vi "PID controlled cooling fan system.vi"() -> ()   [LabVIEW 2024]
panel:
  out "Waveform Chart":cluster{"Temperature (C)":dbl, u8, u8}(graph)
  out "Fan Speed RPM":dbl
  in  "Hardware":bool
  in  "K_d":dbl
  in  "K_i":dbl
  in  "K_p":dbl
  in  "Temperature (C)":dbl
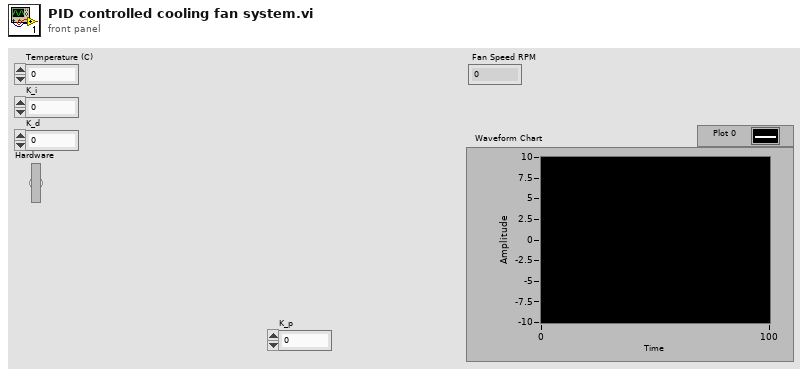
[diagram p1: front panel]
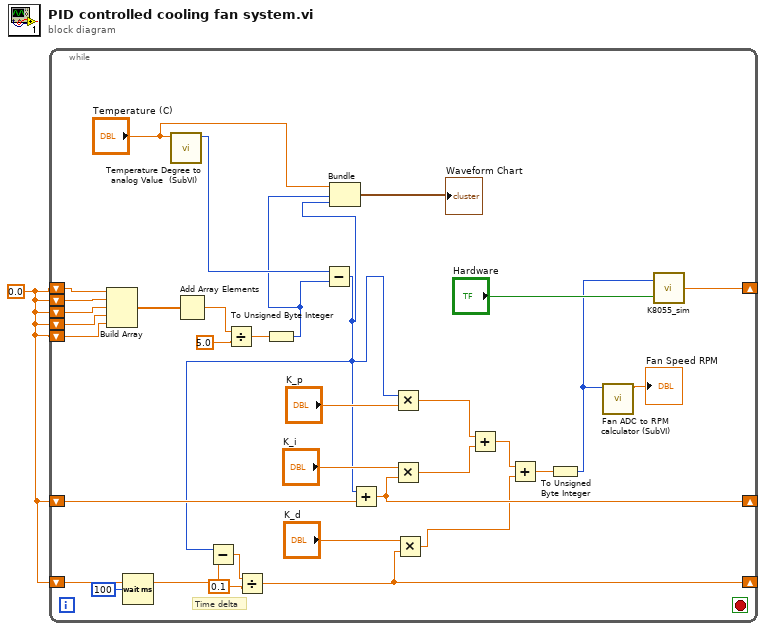
[diagram p0: block diagram]
diagram:
  w1 = 0.0 ("Read temp")
  n1 = while {
    shift-right: [w29] -> _
    shift-left: w1 -> [w34]
    shift-left: w1 -> [w30]
    shift-left: w1 -> [w33]
    shift-left: w1 -> [w32]
    shift-left: w1 -> [w31]
    shift-right: [w19] -> _
    shift-left: w1 -> [w20]
    shift-right: [w6] -> _
    shift-left: w1 -> [w14]
    stop <- _ stop-if-true
    # "Time delta"
    n2 = Build Array(w34, w33, w32, w31, w30) -> (w28:dbl[])
    n3 = Wait (ms)(milliseconds to wait=u32 100) -> ()  [unwired: 1 out]
    n4 = call "Temperature Degree to analog Value  (SubVI).vi"("Temperature (C)"="Temperature (C)") -> ("Temperature Analog Value"=w24:u8)  [unwired: 10 in]
    n5 = Add Array Elements(numeric array=w28) -> (sum=w26:dbl)
    n6 = Divide(x=w26, y=5.0) -> (x/y=w25:dbl)
    n7 = To Unsigned Byte Integer(number=w25) -> (unsigned 8bit integer=w5:u8)
    n8 = Subtract(x=w24, y=w5) -> (x-y=w3:u8)
    n9 = Subtract(x=w3, y=w14) -> (x-y=w13:dbl)
    n10 = Divide(x=w13, y=0.1) -> (x/y=w6:dbl)
    n11 = Bundle("Temperature (C)"="Temperature (C)", w5, w3) -> (→"Waveform Chart":cluster{"Temperature (C)":dbl, u8, u8})  [unwired: 1 in]
    n12 = Add(x=w3, y=w20) -> (x+y=w19:dbl)
    n13 = Multiply(x=w3, y="K_p") -> (x*y=w22:dbl)
    n14 = Multiply(x="K_i", y=w19) -> (x*y=w17:dbl)
    n15 = Multiply(x="K_d", y=w6) -> (x*y=w10:dbl)
    n16 = Add(x=w22, y=w17) -> (x+y=w16:dbl)
    n17 = Add(x=w16, y=w10) -> (x+y=w9:dbl)
    n18 = To Unsigned Byte Integer(number=w9) -> (unsigned 8bit integer=w8:u8)
    n19 = call "Fan ADC to RPM calculator (SubVI).vi"("Fan Speed ADC"=w8) -> ("Fan Speed RPM"=→"Fan Speed RPM":dbl)  [unwired: 10 in]
    n20 = call "K8055_sim.vi"("Hardware"="Hardware", "Fan Speed"=w8) -> ("Read temp"=w29:dbl)
  }
